vi "RC_calibration_ver2.vi"(8 "error in (no error)":errorcluster, 10 "Motors IDs Found":u8[](array[numeric]), 11 "VISA resource name":refnum<visa-resource-name>) -> (0 "error out":errorcluster, 1 "Dynamixel Cycles":T1, 2 "output cluster":T2={"Main Dynamixel Set Data"={"Lower Winch Bound (deg)"=0.0, "Upper Winch Bound (deg)"=1000.0}, "Rudder Dynamixel Set Data"={"Lower Winch Bound (deg)"=30.0, "Upper Winch Bound (deg)"=90.0}, "Jib Dynamixel Set Data"={"Lower Winch Bound (deg)"=0.0, "Upper Winch Bound (deg)"=1000.0}}, 3 "VISA resource name out":refnum<visa-resource-name>)   [LabVIEW 2013]
doc: "Allows the user to set the maximum and minimum points for the sails and center the rudder. Necessary because the Dynamixels can't measure their position along the pulley system.\n\nTakes in the port the Dynamixels are plugged into and the indexes of the motors. Outputs the minimum and maximum points for all three motors and what cycle the motors are at when the code ends along with the port and any errors that occurred."
uses:
  Data/TypeDefs/MotorSetup.ctl
  Data/TypeDefs/DynamixelSetupInfo.ctl
  Data/TypeDefs/DynamixelCycleTracker.ctl
  <instrlib>/Dynamixel Motor/Dynamixel Motor.lvlib
panel:
  in  "Dynamixel Cycles Constant":T1
  in  "Rudder centered?":bool
  in  "Rudder offset":dbl=30.0
  in  "Set Rudder position":dbl=150.0
  out "Rudder position":dbl
  in  "Jib movement 2":dbl
  out "Jib Max Bound":dbl
  out "Jib position\nat max":dbl
  out "Jib rotations to max":i32
  in  "Jib at maximum?":bool
  out "Jib minimum":dbl
  in  "Jib at minimum?":bool
  in  "Jib movement 1":dbl
  in  "Main movement 2":dbl
  out "Max Bound":dbl
  out "Main position\nat max":dbl
  out "Main rotations to max":i32
  in  "Main at maximum?":bool
  out "Main minimum":dbl
  in  "Main at minimum?":bool
  in  "Main movement 1":dbl
  # "TODO: Check labels for main/jib are right"
  # "1. Arrow up/down on main movement 1\n     to have sails move toward all in\n2. When it is as far in as is safe (given \n    pulleys) hit \"Main at minimum\" button"
  # "3. Arrow up/down on main movement 2 \n    to have sails move toward all out\n4. When it is as far out as is safe (given \n    pulleys) hit \"Main at maximum\" button"
  # "5. Arrow up/down on jib movement 1\n     to have sails move toward all in\n6. When it is as far in as is safe (given\n    pulleys) hit \"Jib at minimum\" button"
  # "7. Arrow up/down on jib movement 2 \n    to have sails move toward all out\n8. When it is as far out as is safe (given\n    pulleys) hit \"Jib at maximum\" button"
  # "(as of 4/2/2014)\nSail 1 (main?, right if facing toward bow):\n+ speed goes in, makes position count down (including rotations)\n- speed goes out, makes position count up (including rotations)\nSail 2 (jib?, left if facing toward bow):\n+ speed goes out, makes position count down (including rotations)\n- speed goes in, makes position count up (including rotations)"
  # "9. Change rudder position until it is centered,\n     then hit \"rudder centered\"\n10. Set the offset from rudder center to min/max"
  # "Inputs/outputs you don't need to worry about"
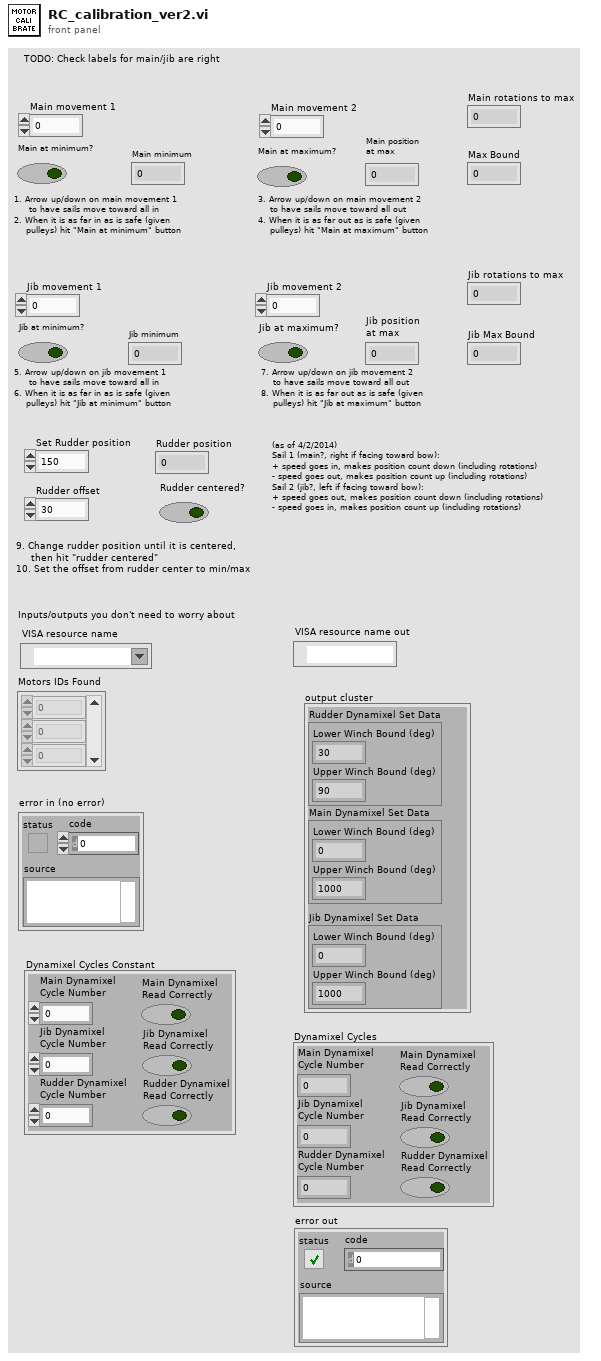
[diagram p1: front panel]
types:
  T1 = typedef "DynamixelCycleTracker.ctl" = cluster{"Main Dynamixel\nCycle Number":i32, "Jib Dynamixel\nCycle Number":i32, "Rudder Dynamixel\nCycle Number":i32, "Main Dynamixel\nRead Correctly":bool, "Jib Dynamixel\nRead Correctly":bool, "Rudder Dynamixel\nRead Correctly":bool}
  T2 = typedef "MotorSetup.ctl" = cluster{"Main Dynamixel Set Data":T3, "Rudder Dynamixel Set Data":T3, "Jib Dynamixel Set Data":T3}
  T3 = typedef "DynamixelSetupInfo.ctl" = cluster{"Lower Winch Bound (deg)":dbl, "Upper Winch Bound (deg)":dbl}
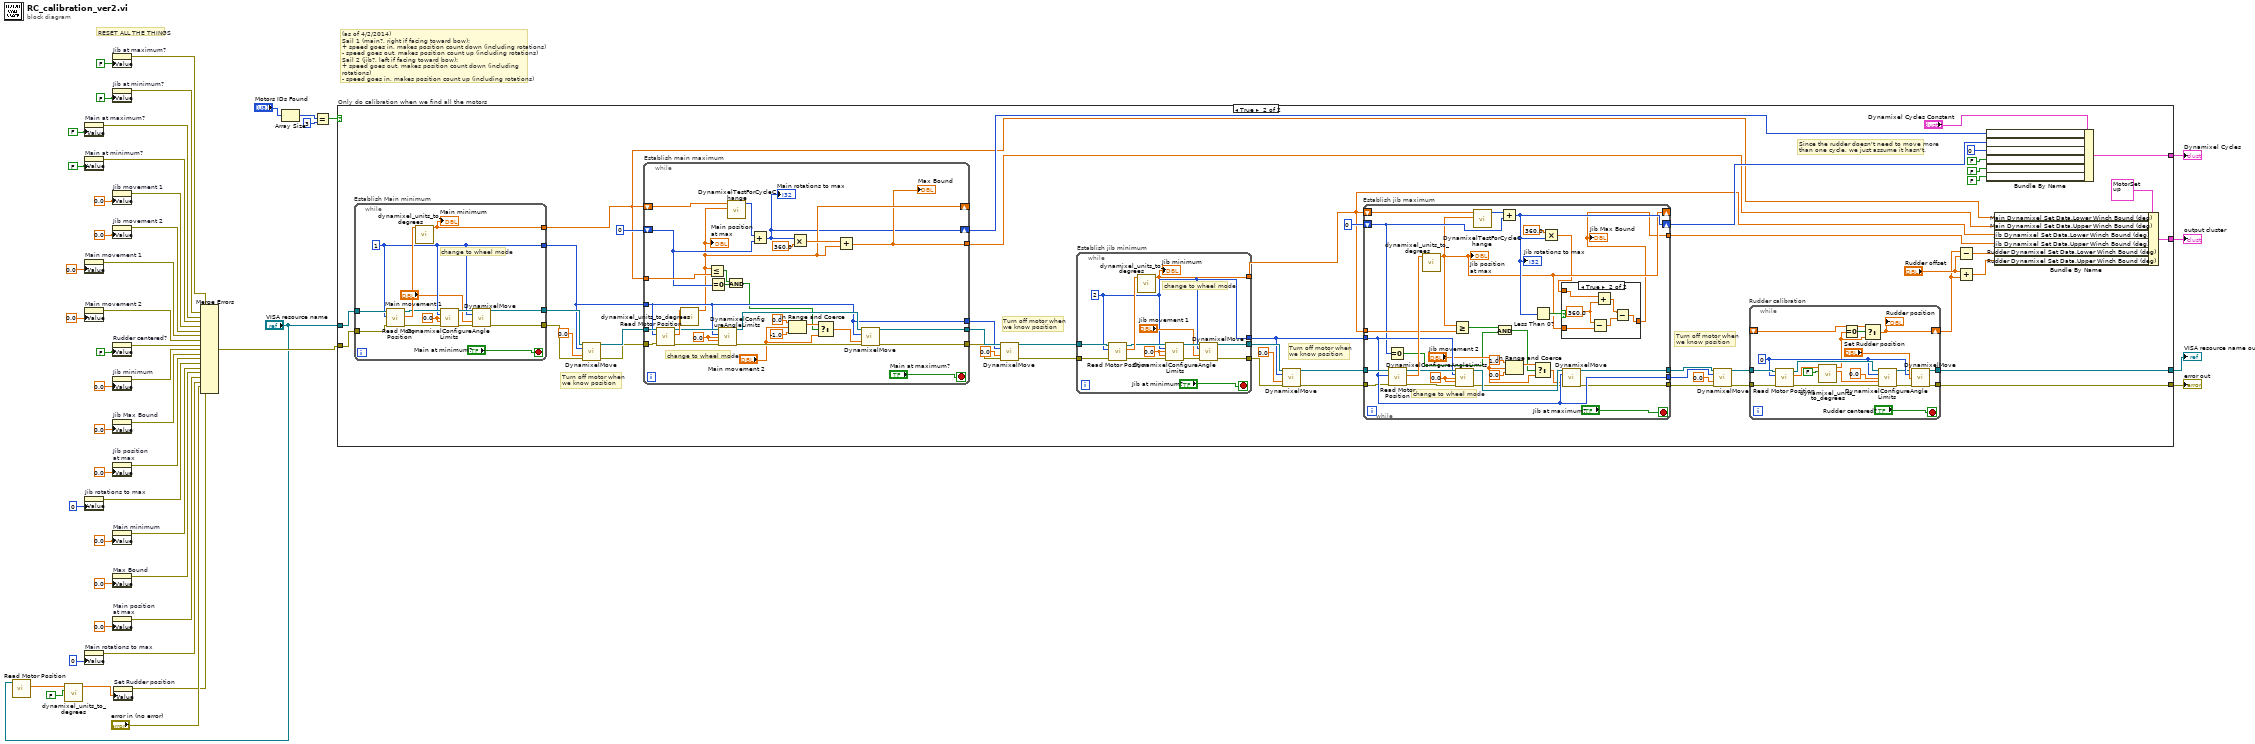
[diagram p0: block diagram]
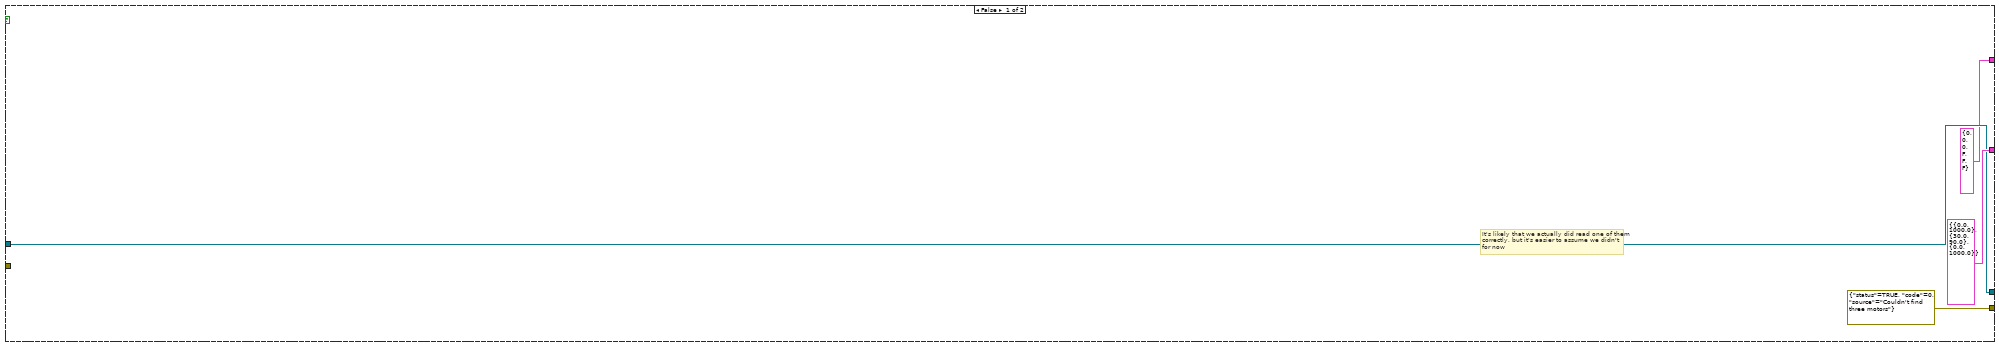
[diagram p2: hidden frame]
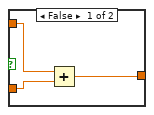
[diagram p3: hidden frame]
diagram:
  # "(as of 4/2/2014)\nSail 1 (main?, right if facing toward bow):\n+ speed goes in, makes position count down (including rotations)\n- speed goes out, makes position count up (including rotations)\nSail 2 (jib?, left if facing toward bow):\n+ speed goes out, makes position count down (including rotations)\n- speed goes in, makes position count up (including rotations)"
  # "RESET ALL THE THINGS"
  n1 = call <instrlib>:"Read Motor Position.vi"("VISA resource name"="VISA resource name") -> ("Position (deg)"=w3:dbl)  [unwired: 8 in, 2 out]
  n2 = call "dynamixel_units_to_degrees.vi"("MX Motor? (T)"=FALSE, "Dynamixel Input"=w3) -> ("Degrees"=w2:dbl)  [unwired: 8 in, 1 out]
  n3 = property on="Main at maximum?" class="Bool (strict)"("Value"=FALSE ("Main at maximum?")) -> (error out=w25:errorcluster)  [unwired: 2 in, 1 out]
  n4 = property on="Main at minimum?" class="Bool (strict)"("Value"=FALSE ("Main at minimum?")) -> (error out=w26:errorcluster)  [unwired: 2 in, 1 out]
  n5 = property on="Main movement 1" class="DigNum (strict)"("Value"=0.0 ("Main movement 1")) -> (error out=w29:errorcluster)  [unwired: 2 in, 1 out]
  n6 = property on="Main movement 2" class="DigNum (strict)"("Value"=0.0 ("Main movement 2")) -> (error out=w30:errorcluster)  [unwired: 2 in, 1 out]
  n7 = property on="Jib rotations to max" class="DigNum (strict)"("Value"=0 ("Jib rotations to max")) -> (error out=w11:errorcluster)  [unwired: 2 in, 1 out]
  n8 = property on="Main rotations to max" class="DigNum (strict)"("Value"=0 ("Main rotations to max")) -> (error out=w7:errorcluster)  [unwired: 2 in, 1 out]
  n9 = property on="Jib at maximum?" class="Bool (strict)"("Value"=FALSE ("Jib at maximum?")) -> (error out=w23:errorcluster)  [unwired: 2 in, 1 out]
  n10 = property on="Jib at minimum?" class="Bool (strict)"("Value"=FALSE ("Jib at minimum?")) -> (error out=w24:errorcluster)  [unwired: 2 in, 1 out]
  n11 = property on="Jib movement 1" class="DigNum (strict)"("Value"=0.0 ("Jib movement 1")) -> (error out=w27:errorcluster)  [unwired: 2 in, 1 out]
  n12 = property on="Jib movement 2" class="DigNum (strict)"("Value"=0.0 ("Jib movement 2")) -> (error out=w28:errorcluster)  [unwired: 2 in, 1 out]
  n13 = property on="Rudder centered?" class="Bool (strict)"("Value"=FALSE ("Rudder centered?")) -> (error out=w31:errorcluster)  [unwired: 2 in, 1 out]
  n14 = property on="Jib minimum" class="DigNum (strict)"("Value"=0.0 ("Jib minimum")) -> (error out=w14:errorcluster)  [unwired: 2 in, 1 out]
  n15 = property on="Jib Max Bound" class="DigNum (strict)"("Value"=0.0 ("Jib offset from\nmin to max")) -> (error out=w13:errorcluster)  [unwired: 2 in, 1 out]
  n16 = property on="Jib position\nat max" class="DigNum (strict)"("Value"=0.0 ("Jib position\nat max")) -> (error out=w12:errorcluster)  [unwired: 2 in, 1 out]
  n17 = property on="Main minimum" class="DigNum (strict)"("Value"=0.0 ("Main minimum")) -> (error out=w10:errorcluster)  [unwired: 2 in, 1 out]
  n18 = property on="Max Bound" class="DigNum (strict)"("Value"=0.0 ("Main offset from\nmin to max")) -> (error out=w9:errorcluster)  [unwired: 2 in, 1 out]
  n19 = property on="Main position\nat max" class="DigNum (strict)"("Value"=0.0 ("Main position\nat max")) -> (error out=w8:errorcluster)  [unwired: 2 in, 1 out]
  n20 = property on="Set Rudder position" class="DigNum (strict)"("Value"=w2) -> (error out=w1:errorcluster)  [unwired: 2 in, 1 out]
  n21 = Merge Errors(w23, w24, w25, w26, w27, w28, w29, w30, w31, w14, w13, w12, w11, w10, w9, w8, w7, "error in (no error)", w1) -> (w32:errorcluster)
  n22 = Array Size(array="Motors IDs Found") -> (size(s)=w48:i32)
  n23 = Equal?(x=w48, y=3) -> (x = y?=w38:bool)
  n24 = case "Only do calibration when we find all the motors" shown="True" w38 {
    tunnel: "VISA resource name" -> [w52 w101]
    tunnel: [T2 {"Main Dynamixel Set Data"={"Lower Winch Bound (deg)"=0.0, "Upper Winch Bound (deg)"=1000.0}, "Rudder Dynamixel Set Data"={"Lower Winch Bound (deg)"=30.0, "Upper Winch Bound (deg)"=90.0}, "Jib Dynamixel Set Data"={"Lower Winch Bound (deg)"=0.0, "Upper Winch Bound (deg)"=1000.0}} ("Dynamixel Bounds Control") w68] -> w49
    tunnel: [w52 w67] -> w45
    tunnel: w32 -> [_ w80]
    tunnel: [errorcluster {"status"=TRUE, "code"=0, "source"="Couldn't find three motors"} ("error out") w66] -> w44
    tunnel: [T1 {"Main Dynamixel\nCycle Number"=0, "Jib Dynamixel\nCycle Number"=0, "Rudder Dynamixel\nCycle Number"=0, "Main Dynamixel\nRead Correctly"=FALSE, "Jib Dynamixel\nRead Correctly"=FALSE, "Rudder Dynamixel\nRead Correctly"=FALSE} ("Dynamixel Cycles Constant") w64] -> w43
    frame False {
      # "It's likely that we actually did read one of them\ncorrectly, but it's easier to assume we didn't \nfor now"
    }
    frame True {
      # "Since the rudder doesn't need to move more\nthan one cycle, we just assume it hasn't."
      # "Turn off motor when \nwe know position"
      # "Turn off motor when \nwe know position"
      # "Turn off motor when \nwe know position"
      # "Turn off motor when \nwe know position"
      n25 = while "Establish Main minimum" {
        tunnel: w101 -> [w186]
        tunnel: [w184] -> w57
        tunnel: [w180] -> w100
        tunnel: [w179] -> w95
        tunnel: w80 -> [w178]
        tunnel: [w175] -> w79
        stop <- "Main at minimum?" stop-if-true
        w182 = 0.0 ("Clockwise Angle Limit (0 deg)")
        w179 = u8 1 ("Motor ID (0)")
        # "change to wheel mode"
        n26 = call <instrlib>:"Read Motor Position.vi"("error in (no error)"=w178, "Motor ID (0)"=w179, "VISA resource name"=w186) -> ("error out"=w177:errorcluster, "Position (deg)"=w185:dbl, "VISA resource name out"=w183:refnum<visa-resource-name>)  [unwired: 6 in]
        n27 = call "dynamixel_units_to_degrees.vi"("Dynamixel Input"=w185) -> ("Degrees"=w184:dbl)  [unwired: 9 in, 1 out]
        "Main minimum" <- w184
        n28 = call "DynamixelConfigureAngleLimits.vi"("VISA resource name"=w183, "Motor ID (0)"=w179, "Clockwise Angle Limit (0 deg)"=w182, "Counter-Clockwise Angle Limit (300 deg)"=w182, "error in (no error)"=w177) -> ("VISA resource name out"=w181:refnum<visa-resource-name>, "error out"=w176:errorcluster)  [unwired: 9 in]
        n29 = call "DynamixelMove.vi"("VISA resource name"=w181, "Motor ID (0)"=w179, "Goal Speed (RPM)"="Main movement 1", "error in (no error)"=w176) -> ("VISA resource name out"=w180:refnum<visa-resource-name>, "error out"=w175:errorcluster)  [unwired: 10 in]
      }
      n30 = call "DynamixelMove.vi"("VISA resource name"=w100, "Motor ID (0)"=w95, "Goal Speed (RPM)"=0.0, "error in (no error)"=w79) -> ("VISA resource name out"=w98:refnum<visa-resource-name>, "error out"=w78:errorcluster)  [unwired: 10 in]
      n31 = while "Establish main maximum" {
        tunnel: w98 -> [w216]
        tunnel: [w211] -> w96
        tunnel: w95 -> [w208]
        tunnel: [w208] -> w85
        tunnel: w78 -> [w207]
        tunnel: [w204] -> w77
        shift-right: [w190] -> _
        shift-left: w57 -> [w203]
        shift-right: [w188] -> w63
        shift-left: 0 ("Dynamixel Cycle Number") -> [w192]
        tunnel: [w189] -> w55
        tunnel: w57 -> [w194]
        stop <- "Main at maximum?" stop-if-true
        w213 = 0.0 ("Clockwise Angle Limit (0 deg)")
        # "change to wheel mode"
        n32 = call <instrlib>:"Read Motor Position.vi"("error in (no error)"=w207, "Motor ID (0)"=w208, "VISA resource name"=w216) -> ("error out"=w206:errorcluster, "Position (deg)"=w215:dbl, "VISA resource name out"=w214:refnum<visa-resource-name>)  [unwired: 6 in]
        n33 = call "dynamixel_units_to_degrees.vi"("Dynamixel Input"=w215) -> ("Degrees"=w190:dbl)  [unwired: 9 in, 1 out]
        "Main position\nat max" <- w190
        n34 = Less Or Equal?(x=w190, y=w194) -> (x <= y?=w193:bool)
        n35 = Equal To 0?(x=w192) -> (x = 0?=w201:bool)
        n36 = call "DynamixelConfigureAngleLimits.vi"("VISA resource name"=w214, "Motor ID (0)"=w208, "Clockwise Angle Limit (0 deg)"=w213, "Counter-Clockwise Angle Limit (300 deg)"=w213, "error in (no error)"=w206) -> ("VISA resource name out"=w212:refnum<visa-resource-name>, "error out"=w205:errorcluster)  [unwired: 9 in]
        n37 = And(x=w193, y=w201) -> (x .and. y?=w197:bool)
        n38 = call "DynamixelTestForCycleChange.vi"("New position (deg)"=w190, "Old position (deg)"=w203) -> ("Dynamixel Cycle Number"=w202:i32)  [unwired: 9 in]
        n39 = Add(x=w202, y=w192) -> (x+y=w188:i32)
        "Main rotations to max" <- w188
        n40 = In Range and Coerce(upper limit=0.0, x="Main movement 2", lower limit=-1.0) -> (coerced(x)=w200:dbl)  [unwired: 1 out]
        n41 = Multiply(x=w188, y=360.0) -> (x*y=w191:dbl)
        n42 = Select(t=w200, s=w197, f="Main movement 2") -> (s? t:f=w195:dbl)
        n43 = Add(x=w191, y=w190) -> (x+y=w189:dbl)
        "Max Bound" <- w189
        n44 = call "DynamixelMove.vi"("VISA resource name"=w212, "Motor ID (0)"=w208, "Goal Speed (RPM)"=w195, "error in (no error)"=w205) -> ("VISA resource name out"=w211:refnum<visa-resource-name>, "error out"=w204:errorcluster)  [unwired: 10 in]
      }
      n45 = call "DynamixelMove.vi"("VISA resource name"=w96, "Motor ID (0)"=w85, "Goal Speed (RPM)"=0.0, "error in (no error)"=w77) -> ("VISA resource name out"=w94:refnum<visa-resource-name>, "error out"=w76:errorcluster)  [unwired: 10 in]
      n46 = while "Establish jib minimum" {
        tunnel: w94 -> [w168]
        tunnel: [w166] -> w92
        tunnel: [w165] -> w56
        tunnel: [w164] -> w90
        tunnel: w76 -> [w163]
        tunnel: [w160] -> w75
        stop <- "Jib at minimum?" stop-if-true
        w170 = 0.0 ("Clockwise Angle Limit (0 deg)")
        w164 = u8 2 ("Motor ID (0)")
        # "change to wheel mode"
        n47 = call <instrlib>:"Read Motor Position.vi"("error in (no error)"=w163, "Motor ID (0)"=w164, "VISA resource name"=w168) -> ("error out"=w162:errorcluster, "Position (deg)"=w172:dbl, "VISA resource name out"=w171:refnum<visa-resource-name>)  [unwired: 6 in]
        n48 = call "dynamixel_units_to_degrees.vi"("Dynamixel Input"=w172) -> ("Degrees"=w165:dbl)  [unwired: 9 in, 1 out]
        "Jib minimum" <- w165
        n49 = call "DynamixelConfigureAngleLimits.vi"("VISA resource name"=w171, "Motor ID (0)"=w164, "Clockwise Angle Limit (0 deg)"=w170, "Counter-Clockwise Angle Limit (300 deg)"=w170, "error in (no error)"=w162) -> ("VISA resource name out"=w169:refnum<visa-resource-name>, "error out"=w161:errorcluster)  [unwired: 9 in]
        n50 = call "DynamixelMove.vi"("VISA resource name"=w169, "Motor ID (0)"=w164, "Goal Speed (RPM)"="Jib movement 1", "error in (no error)"=w161) -> ("VISA resource name out"=w166:refnum<visa-resource-name>, "error out"=w160:errorcluster)  [unwired: 10 in]
      }
      n51 = call "DynamixelMove.vi"("VISA resource name"=w92, "Motor ID (0)"=w90, "Goal Speed (RPM)"=0.0, "error in (no error)"=w75) -> ("VISA resource name out"=w91:refnum<visa-resource-name>, "error out"=w74:errorcluster)  [unwired: 10 in]
      n52 = while "Establish jib maximum" {
        tunnel: w91 -> [w145]
        tunnel: w90 -> [w143]
        tunnel: [w144] -> w88
        tunnel: [w143] -> w87
        tunnel: [w121] -> w54
        tunnel: w74 -> [w142]
        tunnel: [w139] -> w73
        shift-right: [w123] -> _
        shift-left: w56 -> [w138]
        shift-right: [w125] -> w62
        shift-left: 0 -> [w126]
        tunnel: w56 -> [w129]
        stop <- "Jib at maximum?" stop-if-true
        w148 = 0.0 ("Clockwise Angle Limit (0 deg)")
        # "change to wheel mode"
        n53 = Equal To 0?(x=w126) -> (x = 0?=w127:bool)
        n54 = call <instrlib>:"Read Motor Position.vi"("error in (no error)"=w142, "Motor ID (0)"=w143, "VISA resource name"=w145) -> ("error out"=w141:errorcluster, "Position (deg)"=w150:dbl, "VISA resource name out"=w149:refnum<visa-resource-name>)  [unwired: 6 in]
        n55 = call "dynamixel_units_to_degrees.vi"("Dynamixel Input"=w150) -> ("Degrees"=w123:dbl)  [unwired: 9 in, 1 out]
        "Jib position\nat max" <- w123
        n56 = Greater Or Equal?(x=w123, y=w129) -> (x >= y?=w128:bool)
        n57 = call "DynamixelConfigureAngleLimits.vi"("VISA resource name"=w149, "Motor ID (0)"=w143, "Clockwise Angle Limit (0 deg)"=w148, "Counter-Clockwise Angle Limit (300 deg)"=w148, "error in (no error)"=w141) -> ("VISA resource name out"=w147:refnum<visa-resource-name>, "error out"=w140:errorcluster)  [unwired: 9 in]
        n58 = call "DynamixelTestForCycleChange.vi"("New position (deg)"=w123, "Old position (deg)"=w138) -> ("Dynamixel Cycle Number"=w137:i32)  [unwired: 9 in]
        n59 = And(x=w128, y=w127) -> (x .and. y?=w132:bool)
        n60 = Add(x=w137, y=w126) -> (x+y=w125:i32)
        "Jib rotations to max" <- w125
        n61 = In Range and Coerce(upper limit=1.0, x="Jib movement 2", lower limit=0.0) -> (coerced(x)=w135:dbl)  [unwired: 1 out]
        n62 = Select(t=w135, s=w132, f="Jib movement 2") -> (s? t:f=w130:dbl)
        n63 = Less Than 0?(x=w125) -> (x < 0?=w124:bool)
        n64 = Multiply(x=360.0 ("y"), y=w125) -> (x*y=w122:dbl)
        n65 = case shown="True" w124 {
          tunnel: w123 -> [w153 w159]
          tunnel: w122 -> [w152 w156]
          tunnel: [w151 w157] -> w121
          frame False {
            n66 = Add(x=w152, y=w153) -> (x+y=w151:dbl)
          }
          frame True {
            w154 = 360.0 ("x")
            n67 = Subtract(x=w154, y=w159) -> (x-y=w158:dbl)
            n68 = Add(x=w156, y=w154) -> (x+y=w155:dbl)
            n69 = Subtract(x=w155, y=w158) -> (x-y=w157:dbl)
          }
        }
        "Jib Max Bound" <- w121
        n70 = call "DynamixelMove.vi"("VISA resource name"=w147, "Motor ID (0)"=w143, "Goal Speed (RPM)"=w130, "error in (no error)"=w140) -> ("VISA resource name out"=w144:refnum<visa-resource-name>, "error out"=w139:errorcluster)  [unwired: 10 in]
      }
      n71 = call "DynamixelMove.vi"("VISA resource name"=w88, "Motor ID (0)"=w87, "Goal Speed (RPM)"=0.0, "error in (no error)"=w73) -> ("VISA resource name out"=w84:refnum<visa-resource-name>, "error out"=w72:errorcluster)  [unwired: 10 in]
      n72 = while "Rudder calibration" {
        tunnel: w84 -> [w120]
        tunnel: [w116] -> w67
        tunnel: w72 -> [w115]
        tunnel: [w114] -> w66
        shift-right: [w102] -> w69
        shift-left: _ -> [w105]
        stop <- "Rudder centered?" stop-if-true
        w110 = u8 0 ("Motor ID (0)")
        n73 = call <instrlib>:"Read Motor Position.vi"("error in (no error)"=w115, "Motor ID (0)"=w110, "VISA resource name"=w120) -> ("error out"=w108:errorcluster, "Position (deg)"=w119:dbl, "VISA resource name out"=w112:refnum<visa-resource-name>)  [unwired: 6 in]
        n74 = call "dynamixel_units_to_degrees.vi"("MX Motor? (T)"=FALSE, "Dynamixel Input"=w119) -> ("Dynamixel units/cycle"=w111:dbl, "Degrees"=w103:dbl)  [unwired: 8 in]
        n75 = Equal To 0?(x=w103) -> (x = 0?=w104:bool)
        n76 = Select(t=w105, s=w104, f=w103) -> (s? t:f=w102:dbl)
        "Rudder position" <- w102
        n77 = call "DynamixelConfigureAngleLimits.vi"("VISA resource name"=w112, "Motor ID (0)"=w110, "Clockwise Angle Limit (0 deg)"=0.0, "Counter-Clockwise Angle Limit (300 deg)"=w111, "error in (no error)"=w108) -> ("VISA resource name out"=w106:refnum<visa-resource-name>, "error out"=w107:errorcluster)  [unwired: 9 in]
        n78 = call "DynamixelMove.vi"("VISA resource name"=w106, "Motor ID (0)"=w110, "Goal Position (150 deg)"="Set Rudder position", "error in (no error)"=w107) -> ("VISA resource name out"=w116:refnum<visa-resource-name>, "error out"=w114:errorcluster)  [unwired: 10 in]
      }
      n79 = Subtract(x=w69, y="Rudder offset") -> (x-y=w83:dbl)
      n80 = Add(x="Rudder offset", y=w69) -> (x+y=w81:dbl)
      n81 = Bundle By Name(cluster="Dynamixel Cycles Constant", "Main Dynamixel\nCycle Number"=w63, "Jib Dynamixel\nCycle Number"=w62, "Rudder Dynamixel\nCycle Number"=0 ("Rudder Dynamixel\nCycle Number"), "Main Dynamixel\nRead Correctly"=FALSE ("Main Dynamixel\nRead Correctly"), "Jib Dynamixel\nRead Correctly"=FALSE ("Jib Dynamixel\nRead Correctly"), "Rudder Dynamixel\nRead Correctly"=FALSE ("Rudder Dynamixel\nRead Correctly")) -> (w64:T1)
      n82 = Bundle By Name(cluster=T2 {"Main Dynamixel Set Data"={"Lower Winch Bound (deg)"=122.55131964809384, "Upper Winch Bound (deg)"=922.5513196480938}, "Rudder Dynamixel Set Data"={"Lower Winch Bound (deg)"=15.0, "Upper Winch Bound (deg)"=60.0}, "Jib Dynamixel Set Data"={"Lower Winch Bound (deg)"=241.0557184750733, "Upper Winch Bound (deg)"=1041.0557184750733}} ("Dynamixel Bounds Control"), "Main Dynamixel Set Data.Lower Winch Bound (deg)"=w57, "Main Dynamixel Set Data.Upper Winch Bound (deg)"=w55, "Jib Dynamixel Set Data.Lower Winch Bound (deg)"=w56, "Jib Dynamixel Set Data.Upper Winch Bound (deg)"=w54, "Rudder Dynamixel Set Data.Lower Winch Bound (deg)"=w83, "Rudder Dynamixel Set Data.Upper Winch Bound (deg)"=w81) -> (w68:T2)
    }
  }
  "output cluster" <- w49
  "VISA resource name out" <- w45
  "error out" <- w44
  "Dynamixel Cycles" <- w43
